vi "Create Fake Session Reservation.vi"(8 "error in":errorcluster, 10 "session exists":bool=TRUE, 11 "number of sessions":i32=1) -> (0 "error out":errorcluster, 3 "session reservation out":refnum<class "Session Reservation.lvclass">)   [LabVIEW 2020, in "Session Reservation Test Utilities.lvlib"]
uses:
  Session Reservation Test Utilities.lvlib
  Runtime/APIs/Session Management V1/Session Reservation/Session Reservation.lvclass
  Runtime/APIs/Session Management V1/Session Reservation/Data.ctl
  Runtime/APIs/Session Management V1/Session Reservation/Session and Driver Info.ctl
  gRPC/Generated APIs/ni/measurementlink/sessionmanagement/v1/RPC Messages/ni_measurementlink_sessionmanagement_v1_SessionInformation.ctl
  gRPC/Generated APIs/ni/measurementlink/sessionmanagement/v1/RPC Messages/nidevice_grpc_Session.ctl
  gRPC/Generated APIs/ni/measurementlink/sessionmanagement/v1/RPC Messages/ni_measurementlink_sessionmanagement_v1_ChannelMapping.ctl
  Runtime/Sessions/Instrument Sessions/ISession Factory/ISession Factory.lvclass
  Runtime/Sessions/Instrument Sessions/ISession Factory/Initialize and Close Session Behavior.ctl
  Runtime/APIs/Session Management V1/Connection Map/Connection Map.lvclass
  gRPC/Generated APIs/ni/measurementlink/sessionmanagement/v1/RPC Messages/ni_measurementlink_PinMapContext.ctl
  Runtime/APIs/Session Management V1/IReservation Observer/IReservation Observer.lvclass
  Runtime/APIs/Session Management V1/Session Reservation/Group Mapping.ctl
  gRPC/Generated APIs/ni/measurementlink/sessionmanagement/v1/ni.measurementlink.sessionmanagement.v1.api.lvlib
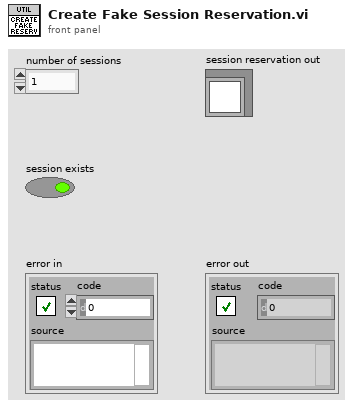
[diagram p1: front panel]
types:
  T1 = typedef "ni.measurementlink.sessionmanagement.v1.api.lvlib/ni_measurementlink_PinMapContext.ctl" = cluster{"pin_map_id":string, "sites":i32[]}
  T2 = typedef "Plug-In SDK Session Management V1 API.lvlib/Session Reservation.lvclass/Data.ctl" = cluster{"session and driver infos":T3[], "pin or relay names":string[], "connection map":refnum<class "Connection Map.lvclass">, "pin map context":T1, "reservation observer":refnum<class "IReservation Observer.lvclass">, "dvr valid":bool, "group mappings":T8}
  T3 = typedef "Plug-In SDK Session Management V1 API.lvlib/Session Reservation.lvclass/Session and Driver Info.ctl" = cluster{"session info":T4, "session":variant, "session factory":refnum<class "ISession Factory.lvclass">, "initialize and close session behavior":T7}
  T4 = typedef "ni.measurementlink.sessionmanagement.v1.api.lvlib/ni_measurementlink_sessionmanagement_v1_SessionInformation.ctl" = cluster{"session":T5, "resource_name":string, "channel_list":string, "instrument_type_id":string, "session_exists":bool, "channel_mappings":T6[]}
  T5 = typedef "ni.measurementlink.sessionmanagement.v1.api.lvlib/nidevice_grpc_Session.ctl" = cluster{"name":string}
  T6 = typedef "ni.measurementlink.sessionmanagement.v1.api.lvlib/ni_measurementlink_sessionmanagement_v1_ChannelMapping.ctl" = cluster{"pin_or_relay_name":string, "site":i32, "channel":string, "multiplexer_resource_name":string, "multiplexer_route":string}
  T7 = typedef "Plug-In SDK Instrument Sessions.lvlib/ISession Factory.lvclass/Initialize and Close Session Behavior.ctl" = enum16{"Initialize and Close", "Attach and Detach", "Initialize and Detach", "Attach and Close"}
  T8 = typedef "Plug-In SDK Session Management V1 API.lvlib/Session Reservation.lvclass/Group Mapping.ctl" = map{string, string[]}
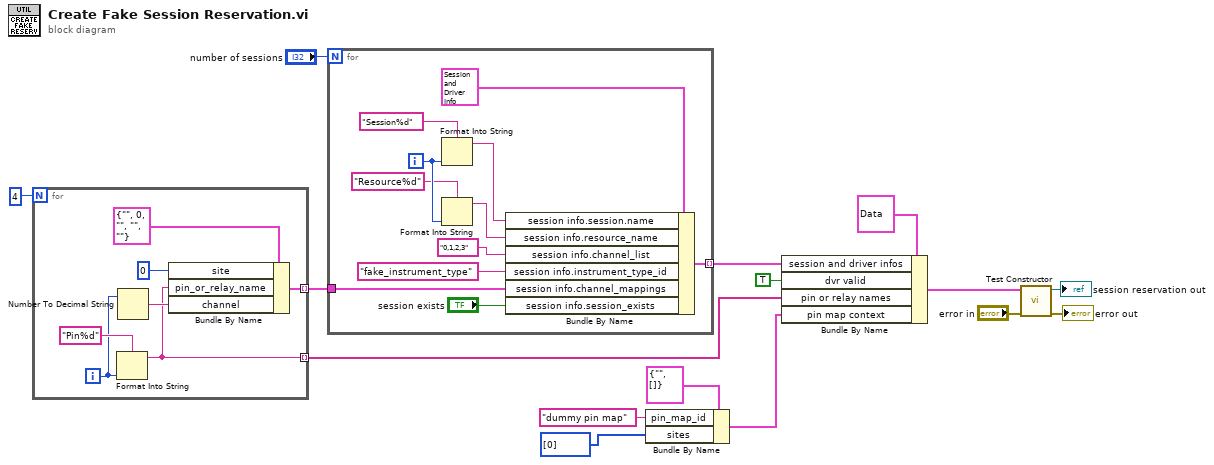
[diagram p0: block diagram]
diagram:
  n1 = for {
    N: 4 -> [_]
    tunnel: [w18] -> w11 mode=indexing
    tunnel: [w17] -> w7 mode=indexing
    i -> [w20]
    n2 = Format Into String(format string="Pin%d", w20) -> (resulting string=w17:string)  [unwired: 2 in, 1 out]
    n3 = Number To Decimal String(number=w20) -> (decimal integer string=w19:string)  [unwired: 1 in]
    n4 = Bundle By Name(cluster=T6 {"pin_or_relay_name"="", "site"=0, "channel"="", "multiplexer_resource_name"="", "multiplexer_route"=""} ("ni_measurementlink_sessionmanagement_v1_ChannelMapping"), "site"=0, "pin_or_relay_name"=w17, "channel"=w19) -> (w18:T6)
  }
  n5 = for {
    N: "number of sessions" -> [_]
    tunnel: w11 -> [w32]
    tunnel: [w31] -> w9 mode=indexing
    i -> [w33]
    n6 = Format Into String(format string="Session%d", w33) -> (resulting string=w27:string)  [unwired: 2 in, 1 out]
    n7 = Format Into String(format string="Resource%d", w33) -> (resulting string=w26:string)  [unwired: 2 in, 1 out]
    n8 = Bundle By Name(cluster=T3 {"session info"={"session"={"name"=""}, "resource_name"="", "channel_list"="", "instrument_type_id"="", "session_exists"=FALSE, "channel_mappings"=[]}, "session"=variant, "session factory"=refnum, "initialize and close session behavior"=enum."Initialize and Close"} ("element"), "session info.session.name"=w27, "session info.resource_name"=w26, "session info.channel_list"="0,1,2,3", "session info.instrument_type_id"="fake_instrument_type", "session info.channel_mappings"=w32, "session info.session_exists"="session exists") -> (w31:T3)
  }
  n9 = Bundle By Name(cluster=T1 {"pin_map_id"="", "sites"=[]} ("pin map context"), "pin_map_id"="dummy pin map", "sites"=i32[] [0]) -> (w1:T1)
  n10 = Bundle By Name(cluster=T2 {"session and driver infos"=[], "pin or relay names"=[], "connection map"=refnum, "pin map context"={"pin_map_id"="", "sites"=[]}, "reservation observer"=refnum, "dvr valid"=FALSE, "group mappings"={}} ("data"), "session and driver infos"=w9, "dvr valid"=TRUE, "pin or relay names"=w7, "pin map context"=w1) -> (w8:T2)
  n11 = call "Test Constructor.vi"("error in"="error in", "data in"=w8) -> ("error out"=→"error out":errorcluster, "session reservation out"=→"session reservation out":refnum<class "Session Reservation.lvclass">)  [unwired: 7 in, 1 out]
